vi "Compute Gated Decay (Fixed Integration Steps).vi"(4 "Non Dirac IRF or non-0 lifetime":bool, 6 "# Steps":ext, 8 "Error In":errorcluster, 9 "IRF Period":dbl, 10 "Gate & Decay Parameters Array":T1[](array[typedef]) {"A" format="%#_4g"; "s" format="%#_4g"; "sF" format="%#_4g"; "sR" format="%#_4g"; "t_i" format="%#_4g"; "t_0" format="%#_4g"; "tau" format="%#_4g"; "T" format="%#_4g"; "W" format="%#_4g"}, 11 "Time Points {t_i}":dbl[](array[numeric])) -> (0 "Error Out":errorcluster, 3 "{F(t_i)}":dbl[](array[numeric]))   [LabVIEW 2019]
uses:
  Gate & Decay Parameters.ctl
  Gate Type.ctl
  IRF Model.ctl
  Graphs/XY Graph/XY Plot Data.ctl
  Arrays/Linear Ramp End Options.ctl
  Compute Gate-IRF Array.vi
  User-defined Gate function.vi
  Compute Gate-IRF Array.vi/66fd7e26-6dd3-4742-9d1f-1742151c5202.vi
  Phasor_Abort Parallel Computation.vi
  T-Periodic Square Gate.vi
  T-Periodic Triangle Gate.vi
  T-Periodic Sawtooth Gate.vi
  <vilib>/Utility/error.llb/Error Cluster From Error Code.vi
  T-Periodic Finite Edge Square Gate.vi
  T-Periodic Finite Edge Tilted Top Square Gate.vi
  Compute 1-Exp Array.vi
  <vilib>/ErrorRing/Error Ring.xnode
  <vilib>/Analysis/2dsp.llb/Integral Method.ctl
  <vilib>/Analysis/NI_AALPro.lvlib
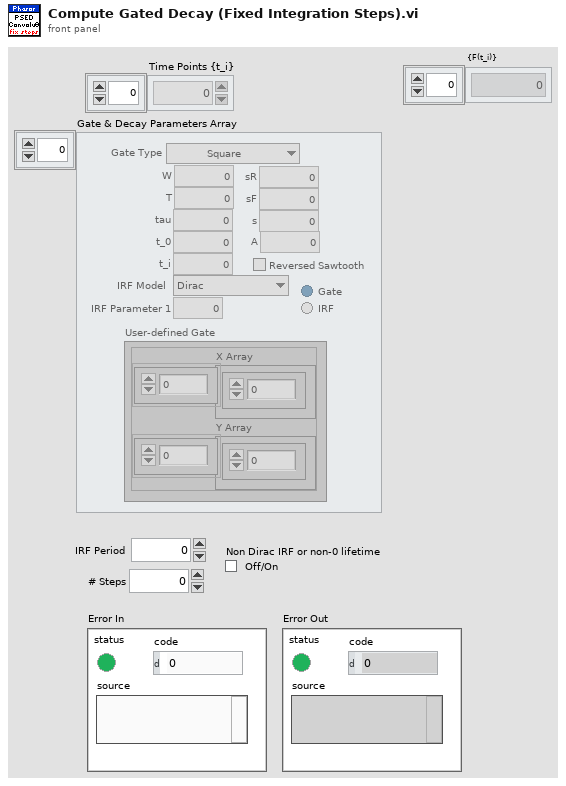
[diagram p1: front panel]
types:
  T1 = typedef "Gate & Decay Parameters.ctl" = cluster{"W":dbl, "T":dbl, "tau":dbl, "t_0":dbl, "Gate Type":T2, "t_i":dbl, "sR":dbl, "sF":dbl, "s":dbl, "Reversed Sawtooth":bool, "IRF Model":T3, "IRF Parameter 1":dbl, "User-defined Gate":T4, "Type of User-defined Function":enum32{"Gate", "IRF"}, "A":dbl}
  T2 = typedef "Gate Type.ctl" = enum16{"Square", "Finite Edge Square", "Finite Edge, Tilted Top Square", "Triangle", "Sawtooth", "User-defined"}
  T3 = typedef "IRF Model.ctl" = enum16{"Dirac", "Exponential"}
  T4 = typedef "XY Plot Data.ctl" = cluster{"X Array":dbl[], "Y Array":dbl[]}
  T5 = typedef "Linear Ramp End Options.ctl" = enum16{"Include Min/Exclude Max", "Exclude Min/Include Max", "Include Both Ends", "Exclude Both Ends"}
  T6 = typedef "NI_AALPro.lvlib/Integral Method.ctl" = i32
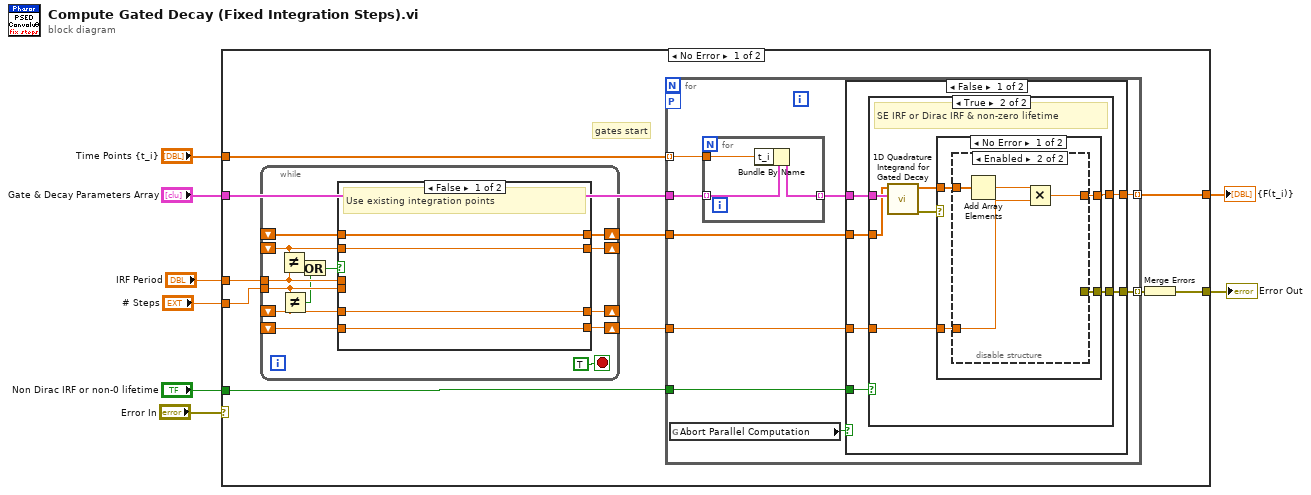
[diagram p0: block diagram]
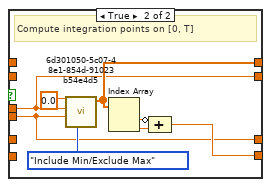
[diagram p2: hidden frame]
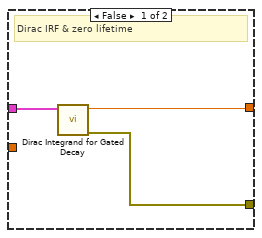
[diagram p3: hidden frame]
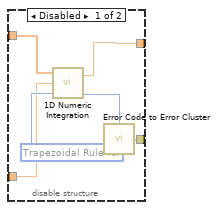
[diagram p4: hidden frame]
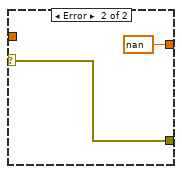
[diagram p5: hidden frame]
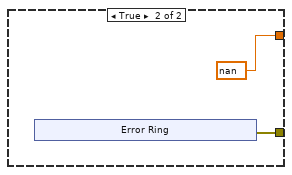
[diagram p6: hidden frame]
diagram:
  n1 = case shown="No Error" "Error In" {
    selector: "Error In" -> [_ w95]
    tunnel: "Non Dirac IRF or non-0 lifetime" -> [w18 _]
    tunnel: "IRF Period" -> [w17 _]
    tunnel: "# Steps" -> [w16 _]
    tunnel: "Time Points {t_i}" -> [w14 _]
    tunnel: "Gate & Decay Parameters Array" -> [w12 _]
    tunnel: [w11 _] -> w3
    tunnel: [w10 w95] -> w2
    frame No Error {
      # "gates start"
      n2 = while {
        tunnel: w17 -> [w30]
        tunnel: w16 -> [w29]
        shift-right: [w32] -> w13
        shift-left: _ -> [w26]
        shift-right: [w20] -> _
        shift-left: _ -> [w19]
        shift-right: [w21] -> _
        shift-left: _ -> [w22]
        shift-right: [w24] -> w9
        shift-left: _ -> [w23]
        stop <- TRUE stop-if-true
        n3 = Not Equal?(x=w22, y=w30) -> (x != y?=w27:bool)
        n4 = Not Equal?(x=w29, y=w19) -> (x != y?=w28:bool)
        n5 = Or(x=w27, y=w28) -> (x .or. y?=w25:bool)
        n6 = case shown="False" w25 {
          tunnel: [w35 w44] -> w24
          tunnel: [w36 w42] -> w32
          tunnel: w30 -> [_ w38]
          tunnel: w29 -> [_ w37]
          tunnel: w26 -> [w36 _]
          tunnel: w23 -> [w35 _]
          tunnel: w22 -> [w34 _]
          tunnel: [w34 w38] -> w21
          tunnel: [w33 w37] -> w20
          tunnel: w19 -> [w33 _]
          frame False {
            # "Use existing integration points"
          }
          frame True {
            # "Compute integration points on [0, T]"
            n7 = call "6d301050-5c07-48e1-854d-91023b54e4d5.vi"("Options"=Linear_Ramp_End_Options."Include Min/Exclude Max", "# Steps (1)"=w37, "End (1)"=w38, "Start (0)"=0.0) -> ("Ramp"=w42:ext[])  [unwired: 5 in, 2 out]
            n8 = Index Array(array=w42) -> (element #1=w41:ext, element #2=w43:ext)  [unwired: 2 in]
            n9 = Compound Arithmetic op=ADD(invert w41, w43) -> (w44:ext)
          }
        }
      }
      n10 = for {
        tunnel: w12 -> [w53]
        tunnel: w14 -> [w47] mode=indexing
        tunnel: w13 -> [w51]
        tunnel: [w50] -> w11 mode=indexing
        tunnel: w9 -> [w49]
        workers-P: _ -> [_]
        tunnel: [w48] -> w15 mode=indexing
        tunnel: w18 -> [w46]
        n11 = global read "Phasor_Abort Parallel Computation.vi" "Abort Parallel Computation"() -> (w45:bool)
        n12 = for {
          tunnel: w53 -> [w56] mode=indexing
          tunnel: [w55] -> w52 mode=indexing
          tunnel: w47 -> [w54]
          n13 = Bundle By Name(cluster=w56, "t_i"=w54) -> (w55:T1)
        }
        n14 = case shown="False" w45 {
          tunnel: w52 -> [w62 _]
          tunnel: w51 -> [w61 _]
          tunnel: [w60 nan ("result")] -> w50
          tunnel: w49 -> [w59 _]
          tunnel: [w58 w89] -> w48
          tunnel: w46 -> [w57 _]
          frame False {
            n15 = case shown="True" w57 {
              tunnel: w62 -> [w65 w72]
              tunnel: w61 -> [_ w70]
              tunnel: [w64 w69] -> w60
              tunnel: w59 -> [_ w68]
              tunnel: [w63 w66] -> w58
              frame False {
                # "Dirac IRF & zero lifetime"
                n16 = call "Dirac Integrand for Gated Decay.vi"("data"=w65) -> ("Error Out"=w63:errorcluster, "F(X)"=w64:dbl)  [unwired: 9 in]
              }
              frame True {
                # "SE IRF or Dirac IRF & non-zero lifetime"
                n17 = call "1D Quadrature Integrand for Gated Decay.vi"("data"=w72, "X"=w70) -> ("Error Out"=w67:errorcluster, "F(X)"=w71:dbl[])  [unwired: 8 in]
                n18 = case shown="No Error" w67 {
                  selector: w67 -> [_ w88]
                  tunnel: w71 -> [w76 _]
                  tunnel: [w75 nan ("result")] -> w69
                  tunnel: w68 -> [w74 _]
                  tunnel: [w73 w88] -> w66
                  frame No Error {
                    n19 = disable-structure shown="Enabled" {
                      disable-tunnel: w76 -> [w81 w86]
                      disable-tunnel: [w80 w83] -> w75
                      disable-tunnel: w74 -> [w79 w84]
                      disable-tunnel: [w77 _] -> w73
                      frame Disabled {
                        w82 = T6 0 items=["Trapezoidal Rule", "Simpson's Rule", "Simpson's 3/8 Rule", "Bode Rule"] ("integration method")
                        n20 = call <vilib>:"1D Numeric Integration.vi"("integration method"=w82, "dt"=w79, "Input Array"=w81) -> ("error"=w78:i32, "result"=w80:dbl)
                        n21 = call "Error Code to Error Cluster.vi"("Error Code"=w78) -> ("Error Out"=w77:errorcluster)  [unwired: 14 in]
                      }
                      frame Enabled {
                        n22 = Add Array Elements(numeric array=w86) -> (sum=w85:dbl)
                        n23 = Multiply(x=w85, y=w84) -> (x*y=w83:ext)
                      }
                    }
                  }
                  frame Error {
                  }
                }
              }
            }
          }
          frame True {
            n24 = xnode "Error Ring"() -> ("error out"=w89:errorcluster)
          }
        }
      }
      n25 = Merge Errors(w15) -> (w10:errorcluster)
    }
    frame Error {
    }
  }
  "{F(t_i)}" <- w3
  "Error Out" <- w2
